vi "Day 11.2 - sync flash.vi"(11 "input":string[](array[string])) -> (3 "output":i32)   [LabVIEW 2021]
panel:
  out "No of flashes":i32
  out "x > y? 3":bool[][](array[boolean])
  out "Numeric 2":i32
  out "Cycle":i32
  out "x > y? 2":bool[][](array[boolean])
  out "Octopus Energy Levels 2":i32[][](array[numeric])
  out "Flash this cycle":bool[][](array[boolean])
  out "Octopus Energy Levels":i32[][](array[numeric])
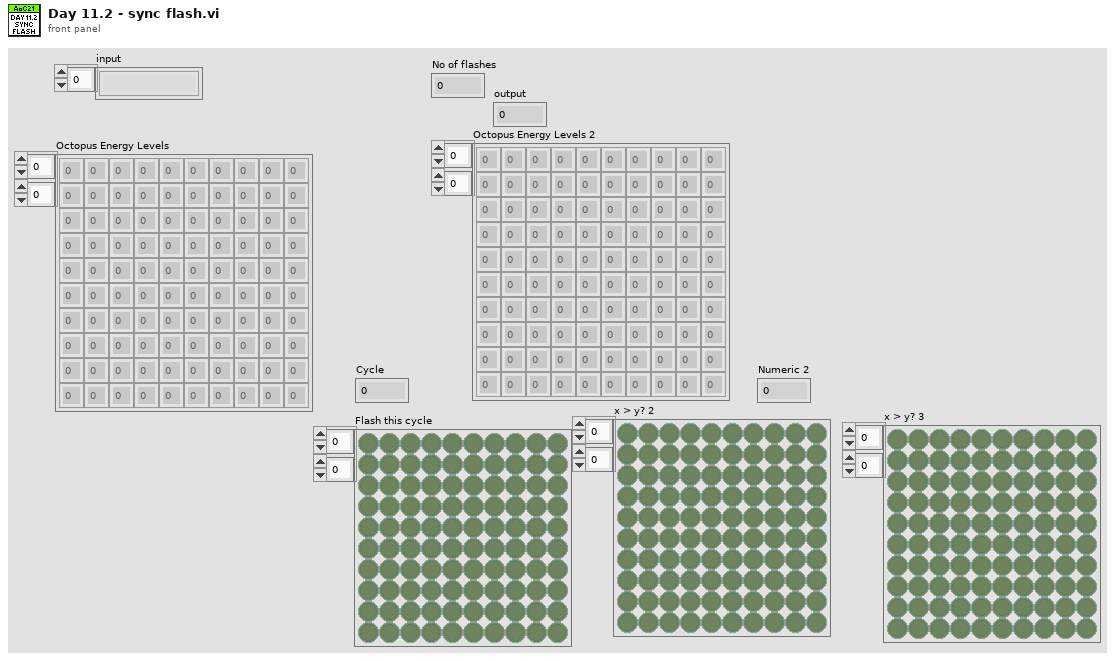
[diagram p1: front panel]
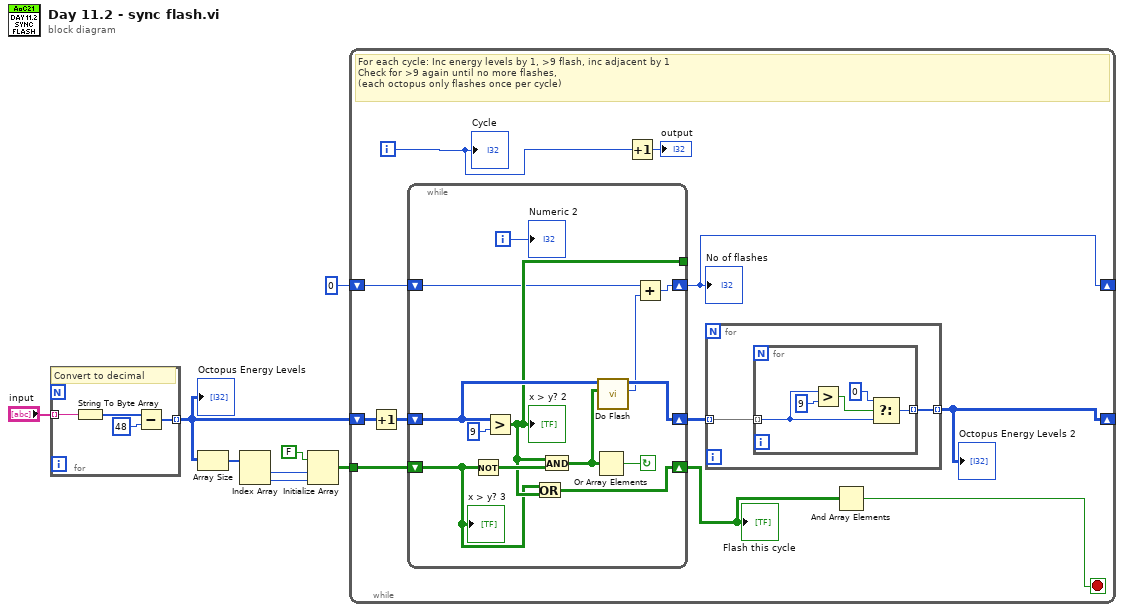
[diagram p0: block diagram]
diagram:
  n1 = for {
    tunnel: "input" -> [w12] mode=indexing
    tunnel: [w9] -> w7 mode=indexing
    # "Convert to decimal"
    n2 = String To Byte Array(string=w12) -> (unsigned byte array=w11:u8[])
    n3 = Subtract(x=w11, y=48) -> (x-y=w9:i32[])
  }
  "Octopus Energy Levels" <- w7
  n4 = Array Size(array=w7) -> (size(s)=w5:i32[])
  n5 = Index Array(array=w5) -> (element #1=w4:i32, element #2=w3:i32)  [unwired: 2 in]
  n6 = Initialize Array(FALSE, w4, w3) -> (w2:bool[][])
  n7 = while {
    tunnel: w2 -> [w21]
    shift-right: [w19] -> _
    shift-left: w7 -> [w23]
    shift-right: [w17] -> _
    shift-left: 0 -> [w18]
    i -> [w14]
    stop <- w15 stop-if-true
    # "For each cycle: Inc energy levels by 1, >9 flash, inc adjacent by 1\nCheck for >9 again until no more flashes, \n(each octopus only flashes once per cycle)"
    n8 = Increment(x=w23) -> (x+1=w22:i32[][])
    n9 = while {
      shift-right: [w42] -> w16
      shift-left: w21 -> [w35]
      shift-right: [w40] -> w20
      shift-left: w22 -> [w41]
      tunnel: [w36] -> _
      shift-right: [w32] -> w17
      shift-left: w18 -> [w31]
      i -> [w37]
      stop <- w38 continue-if-true
      n10 = Not(x=w35) -> (.not. x?=w39:bool[][])
      n11 = Greater?(x=w41, y=9) -> (0:w36:bool[][])
      "x > y? 2" <- w36
      n12 = Or(x=w35, y=w36) -> (x .or. y?=w42:bool[][])
      n13 = And(x=w36, y=w39) -> (x .and. y?=w34:bool[][])
      n14 = Or Array Elements(Boolean array=w34) -> (logical OR=w38:bool)
      n15 = call "Do Flash.vi"("x > y?"=w34, "Octopus Energy Levels in"=w41) -> ("No of flashes"=w33:i32, "Octopus Energy Levels out"=w40:i32[][])  [unwired: 8 in]
      n16 = Add(x=w31, y=w33) -> (x+y=w32:i32)
      "Numeric 2" <- w37
      "x > y? 3" <- w35
    }
    "Flash this cycle" <- w16
    "No of flashes" <- w17
    n17 = Increment(x=w14) -> (x+1=→"output":i32)
    n18 = for {
      tunnel: w20 -> [w25] mode=indexing
      tunnel: [w24] -> w19 mode=indexing
      n19 = for {
        tunnel: w25 -> [w28] mode=indexing
        tunnel: [w26] -> w24 mode=indexing
        n20 = Greater?(x=w28, y=9) -> (0:w29:bool)
        n21 = Select(t=0, s=w29, f=w28) -> (s? t:f=w26:i32)
      }
    }
    "Octopus Energy Levels 2" <- w19
    n22 = And Array Elements(Boolean array=w16) -> (logical AND=w15:bool)
    "Cycle" <- w14
  }
